vi "Parse DB.vi"(8 "error in (no error)":errorcluster, 11 "Path in":path=path "C:/work/SE/Opportunities/2012/Pilatus/201210/TestXMLs/Receiver.xml") -> (0 "error out":errorcluster, 3 "channels":T1 {"speed" items=["OWL429_HIGH_SPEED_CHANNEL", "OWL429_LOW_SPEED_CHANNEL"]; "Labels"."scheduleBuildUnit" items=["Millisecond", "Microsecond"]})   [LabVIEW 2016, in "Ballard Arinc-429 System Explorer.lvlib"]
uses:
  Ballard Arinc-429 System Explorer.lvlib
  Controls/Ballard_Label.ctl
  Controls/Ballard_Channel.ctl
  Controls/Ballard_Channel Array.ctl
  Controls/ARINCParam.ctl
  Controls/Ballard_Word.ctl
  Shared/Controls and Global/TransferType.ctl
  Shared/Ballard Arinc-429 Shared.lvlib
  Controls/Channel_direction.ctl
  Controls/Channel Speed.ctl
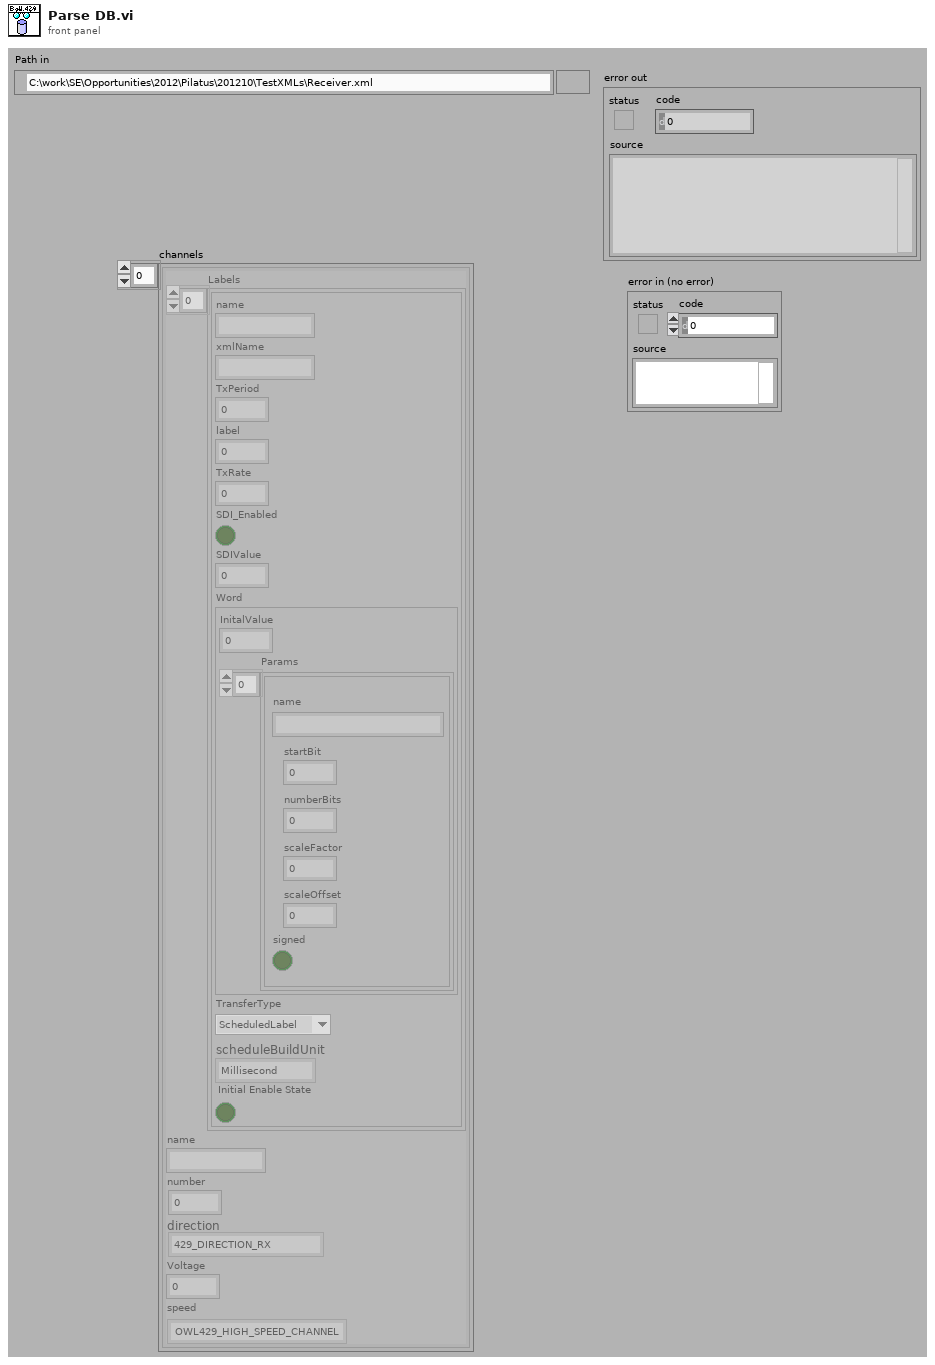
[diagram p1: front panel]
types:
  T1 = typedef "Ballard Arinc-429 System Explorer.lvlib/Ballard_Channel Array.ctl" = T2[]
  T2 = typedef "Ballard Arinc-429 System Explorer.lvlib/Ballard_Channel.ctl" = cluster{"Labels":T3[], "name":string, "number":u8, "direction":T7, "Voltage":dbl, "speed":T8}
  T3 = typedef "Ballard Arinc-429 System Explorer.lvlib/Ballard_Label.ctl" = cluster{"name":string, "xmlName":string, "TxPeriod":u32, "label":u32, "TxRate":dbl, "SDI_Enabled":bool, "SDIValue":u8, "Word":T4, "TransferType":T6, "scheduleBuildUnit":i32, "Initial Enable State":bool}
  T4 = typedef "Ballard Arinc-429 System Explorer.lvlib/Ballard_Word.ctl" = cluster{"InitalValue":u32, "Params":T5[]}
  T5 = typedef "Ballard Arinc-429 System Explorer.lvlib/ARINCParam.ctl" = cluster{"name":string, "startBit":i32, "numberBits":i32, "scaleFactor":dbl, "scaleOffset":dbl, "signed":bool}
  T6 = typedef "Ballard Arinc-429 Shared.lvlib/TransferType.ctl" = enum16{"ScheduledLabel", "Acyclic", "Block", "Strobe"}
  T7 = typedef "Ballard Arinc-429 System Explorer.lvlib/Channel_direction.ctl" = enum16{"429_DIRECTION_RX", "429_DIRECTION_TX"}
  T8 = typedef "Ballard Arinc-429 System Explorer.lvlib/Channel Speed.ctl" = i32
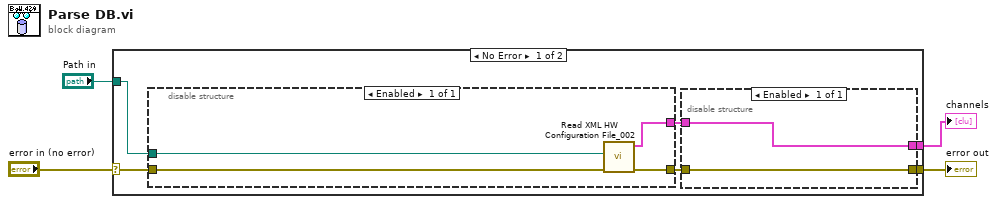
[diagram p0: block diagram]
diagram:
  n1 = case shown="No Error" "error in (no error)" {
    selector: "error in (no error)" -> [w10 w17]
    tunnel: "Path in" -> [w5 _]
    tunnel: [w7 w17] -> w2
    tunnel: [w8 _] -> w1
    frame No Error {
      n2 = disable-structure shown="Enabled" {
        disable-tunnel: w10 -> [w13]
        disable-tunnel: [w16] -> w9
        disable-tunnel: [w15] -> w6
        disable-tunnel: w5 -> [w14]
        frame Enabled {
          n3 = call "Read XML HW Configuration File_002.vi"("error in (no error)"=w13, "XML Configuration File Path"=w14) -> ("error IO"=w16:errorcluster, "channels"=w15:T1)  [unwired: 8 in]
        }
      }
      n4 = disable-structure shown="Enabled" {
        disable-tunnel: w9 -> [w12]
        disable-tunnel: [w11] -> w8
        disable-tunnel: [w12] -> w7
        disable-tunnel: w6 -> [w11]
        frame Enabled {
        }
      }
    }
    frame Error {
    }
  }
  "error out" <- w2
  "channels" <- w1
